vi "isEmpty.vi"(8 "error in (no error)":errorcluster, 11 "xwpfRun in":refnum<class "xwpfRun.lvclass">) -> (0 "error out":errorcluster, 2 "IsEmpty":bool, 3 "xwpfRun out":refnum<class "xwpfRun.lvclass">)   [LabVIEW 2017, in "Word_Specific.lvlib" / "xwpfRun.lvclass"]
uses:
  xwpfRun.lvclass
  xwpfRun.lvclass/xwpfRun.ctl
  C:/Users/Neo/Desktop/Dev_Tools_BR/LabVIEW_NPOI/src/lib/NPOI 2.1.1/NPOI.OOXML.dll
  lib/NPOI 2.1.1/NPOI.OOXML.dll
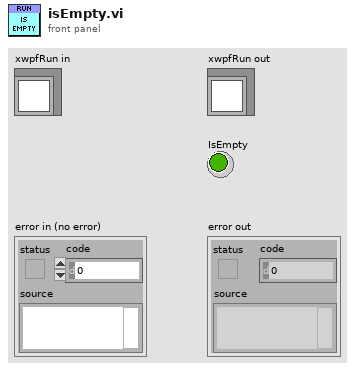
[diagram p1: front panel]
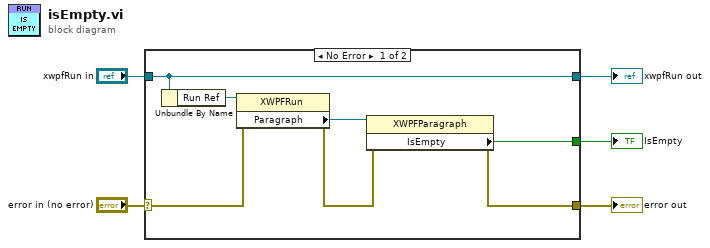
[diagram p0: block diagram]
diagram:
  n1 = case shown="No Error" "error in (no error)" {
    selector: "error in (no error)" -> [w9 w14]
    tunnel: [w6 w14] -> w4
    tunnel: [w12 w13] -> w2
    tunnel: "xwpfRun in" -> [w12 w13]
    tunnel: [w7 _] -> w1
    frame No Error {
      n2 = Unbundle By Name(w12) -> ("Run Ref"=w11:refnum<k24>)
      n3 = property class="XWPFRun"(reference=w11, error in=w9) -> (error out=w8:errorcluster, "Paragraph"=w10:refnum<k24>)  [unwired: 1 out]
      n4 = property class="XWPFParagraph"(reference=w10, error in=w8) -> (error out=w6:errorcluster, "IsEmpty"=w7:bool)  [unwired: 1 out]
    }
    frame Error {
    }
  }
  "error out" <- w4
  "xwpfRun out" <- w2
  "IsEmpty" <- w1
